vi "Live_Update_Value_indicator.vi"(0 "Value Indicators Ref":refnum<vi>[](array[refnum]), 1 "Array in":u16[](array[numeric]), 3 "error out":errorcluster) -> ()   [LabVIEW 2017]
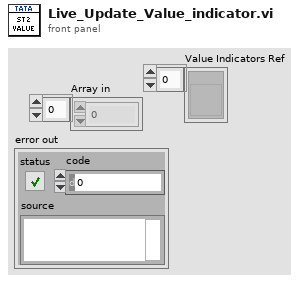
[diagram p1: front panel]
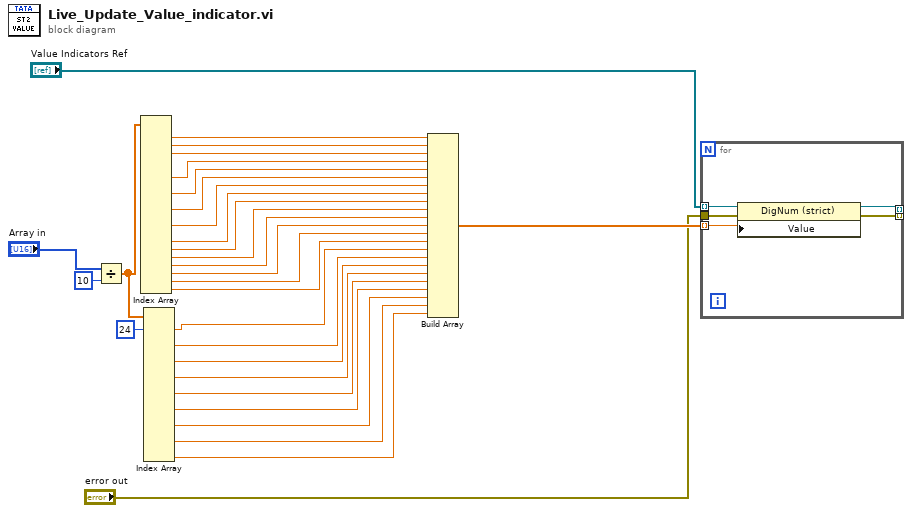
[diagram p0: block diagram]
diagram:
  n1 = Divide(x="Array in", y=10 ("Numeric 2")) -> (x/y=w7:dbl[])
  n2 = Index Array(array=w7) -> (element #1=w8:dbl, element #2=w9:dbl, element #3=w10:dbl, element #6=w11:dbl, element #8=w12:dbl, element #10=w13:dbl, element #12=w14:dbl, element #14=w15:dbl, element #15=w16:dbl, element #16=w17:dbl, element #17=w18:dbl, element #18=w19:dbl, element #19=w20:dbl, element #20=w21:dbl)  [unwired: 20 in, 6 out]
  n3 = Index Array(array=w7, index #1=24 ("index")) -> (element #1=w22:dbl, element #3=w23:dbl, element #5=w24:dbl, element #7=w25:dbl, element #9=w26:dbl, element #11=w27:dbl, element #13=w28:dbl, element #15=w29:dbl, element #17=w30:dbl)  [unwired: 16 in, 8 out]
  n4 = Build Array(w8, w9, w10, w11, w12, w13, w14, w15, w16, w17, w18, w19, w20, w21, w22, w23, w24, w25, w26, w27, w28, w29, w30) -> (w3:dbl[])
  n5 = for {
    tunnel: "Value Indicators Ref" -> [w35] mode=indexing
    tunnel: w3 -> [w34] mode=indexing
    tunnel: "error out" -> [w33]
    tunnel: [w32] -> _ mode=indexing
    tunnel: [w31] -> _ mode=indexing
    n6 = property class="DigNum (strict)"(reference=w35, error in=w33, "Value"=w34) -> (reference out=w31:refnum<vi>, error out=w32:errorcluster)
  }
